vi "XYZ-2.vi"() -> ()   [LabVIEW 2010]
uses:
  <vilib>/Utility/error.llb/DialogType.ctl
  <vilib>/DAQmx/write.llb/DAQmx Write (Analog DBL 1Chan 1Samp).vi
  <vilib>/DAQmx/create/channels.llb/DAQmx Create Channel (AO-Voltage-Basic).vi
  <vilib>/daqmx/miscellaneous.llb/DAQmx Fill In Error Info.vi
  Instance           2 20Saved   XYZ 3.6.2.01 .vi
  Instance           5 20Saved   XYZ 3.6.2.01 .vi
  Instance           7 20Saved   XYZ 3.6.2.01 .vi
  Instance           8 20Saved   XYZ 3.6.2.01 .vi
  <vilib>/Utility/file.llb/Write To Spreadsheet File (DBL).vi
  Instance          10 20Saved   XYZ 3.6.2.01 .vi
  Instance          14 20Saved   XYZ 3.6.2.01 .vi
  Instance          11 20Saved   XYZ 3.6.2.01 .vi
  <vilib>/measure/NI_MABase.lvlib
panel:
  in  "save":bool
  out "pos Z":dbl=100.0
  in  "Return Z":bool
  out "Pos Z inv":dbl
  in  "Go to Z":dbl
  in  "R Z":bool
  out "?":bool
  in  "# steps z":dbl
  in  "Amp inv Z":dbl=2.0
  out "Pos Y inv":dbl
  out "Pos z":dbl=1.0
  in  "Max Z":dbl=1.0
  in  "Ampl Z":dbl=2.0
  in  "R Y":bool
  out "?":bool
  in  "Ampl Y Inv":dbl=2.5
  in  "# steps Y":dbl
  out "Pos Y inv":dbl
  out "Pos Y":dbl=1.0
  in  "Max Y":dbl=1.0
  in  "Ampl Y":dbl=2.5
  in  "R X":bool
  out "?":bool
  in  "Ampl X Inv":dbl=2.5
  in  "# steps x":dbl
  out "Pos X inv":dbl
  out "Pos X":dbl=1.0
  in  "Max X":dbl=1.0
  in  "Ampl X":dbl=2.5
  out "?":bool=TRUE
  out "?":bool=TRUE
  in  "Forward":bool=TRUE
  in  "Return Y":bool
  out "pos Y INV":dbl
  in  "Go to Y":dbl
  out "pos Y":dbl=100.0
  in  "Return X":bool
  out "pos X":dbl=100.0
  out "Pos X INV":dbl=543.0
  in  "Go to X":dbl
  in  "MAIN":path=path "C:/Users/John Markert/Desktop/main data.lvm"
  in  "?":bool
  out "Data":dbl[][](array[numeric])=[[0.0, 0.0, 0.0, 4.53e-05, 0.0]]
  out "Matrix 5 x":dbl=1.0
  # "[X,R]"
  # "[Y,0]"
  # "Y"
  # "Z"
  # "X"
  # "Max _ # of groupings\nof # of steps pulses each"
  # "Backwards"
  # "Lock-in ON"
  # "DC Volt ON"
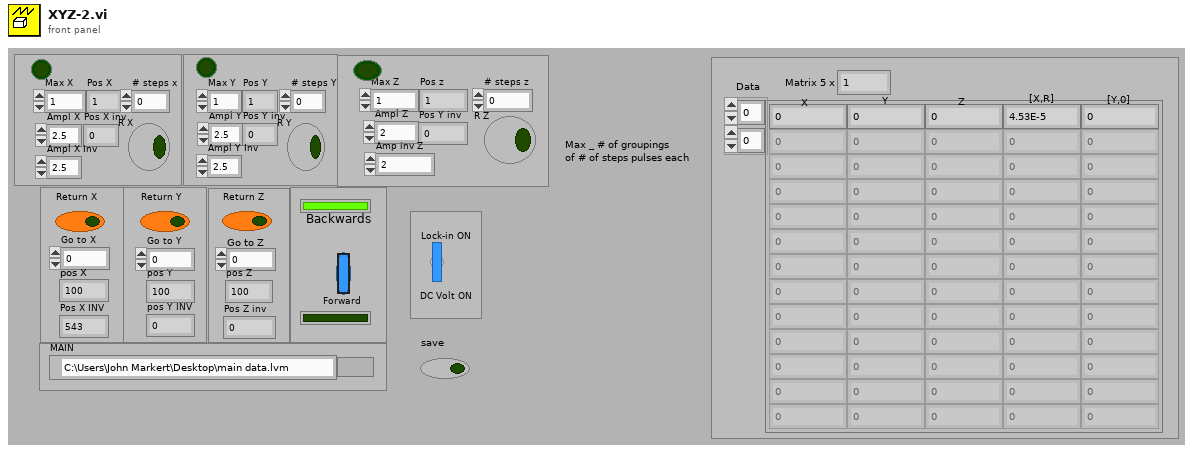
[diagram p1: front panel]
types:
  T1 = typedef "DialogType.ctl" = u16
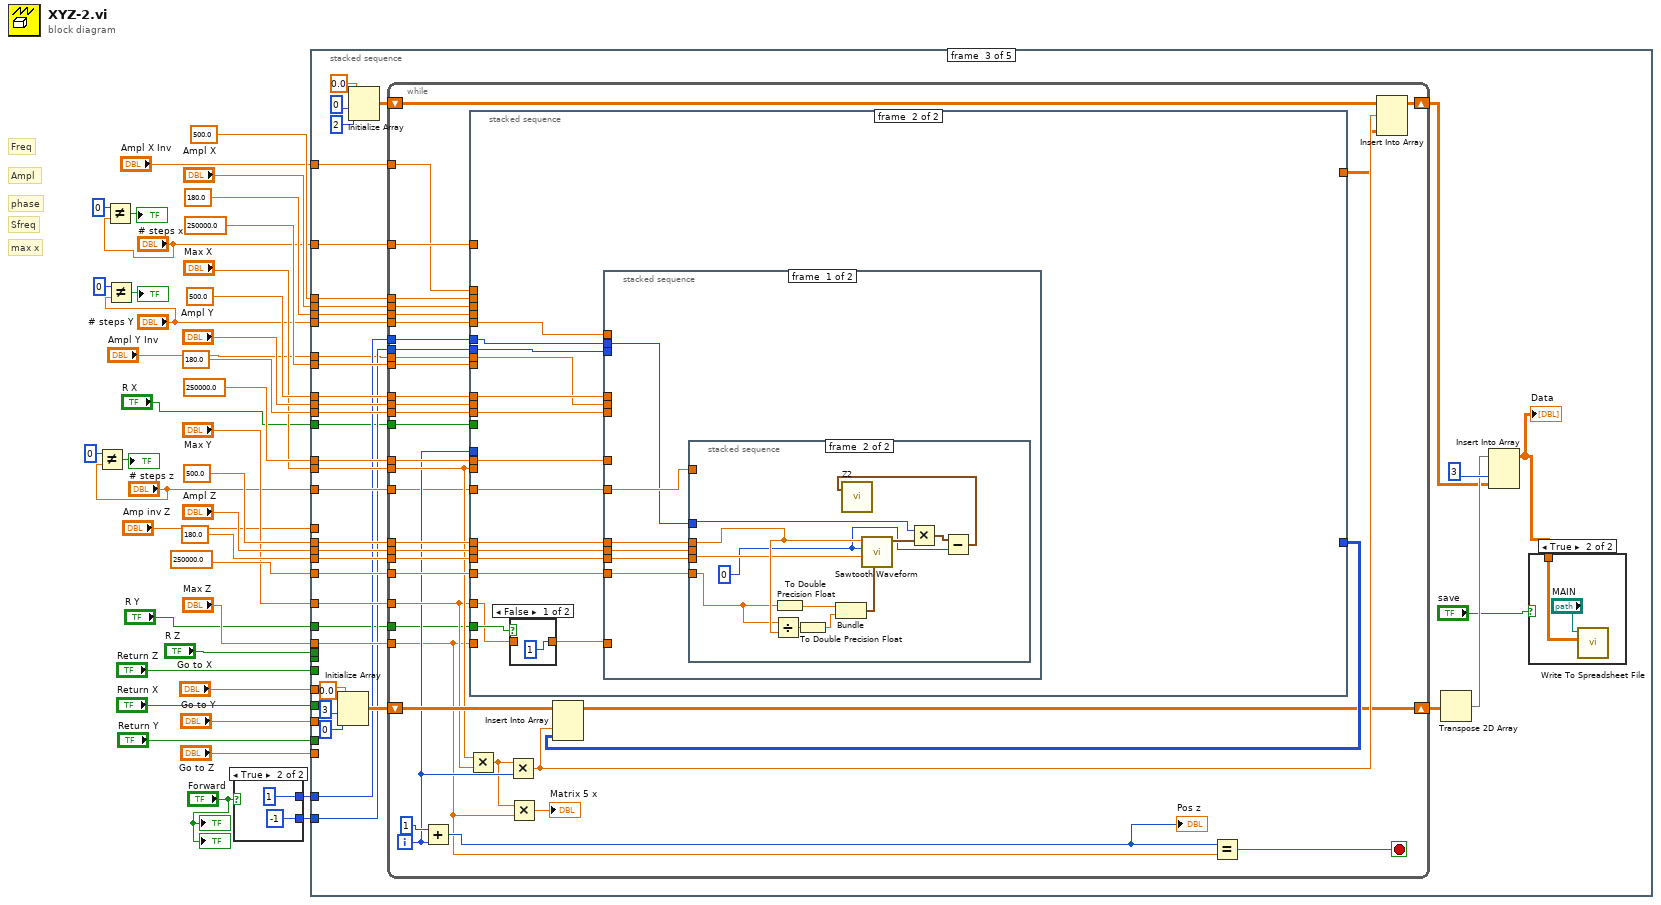
[diagram p0: block diagram]
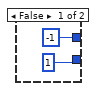
[diagram p2: hidden frame]
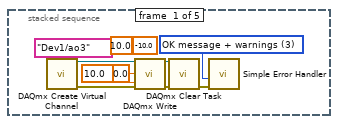
[diagram p3: hidden frame]
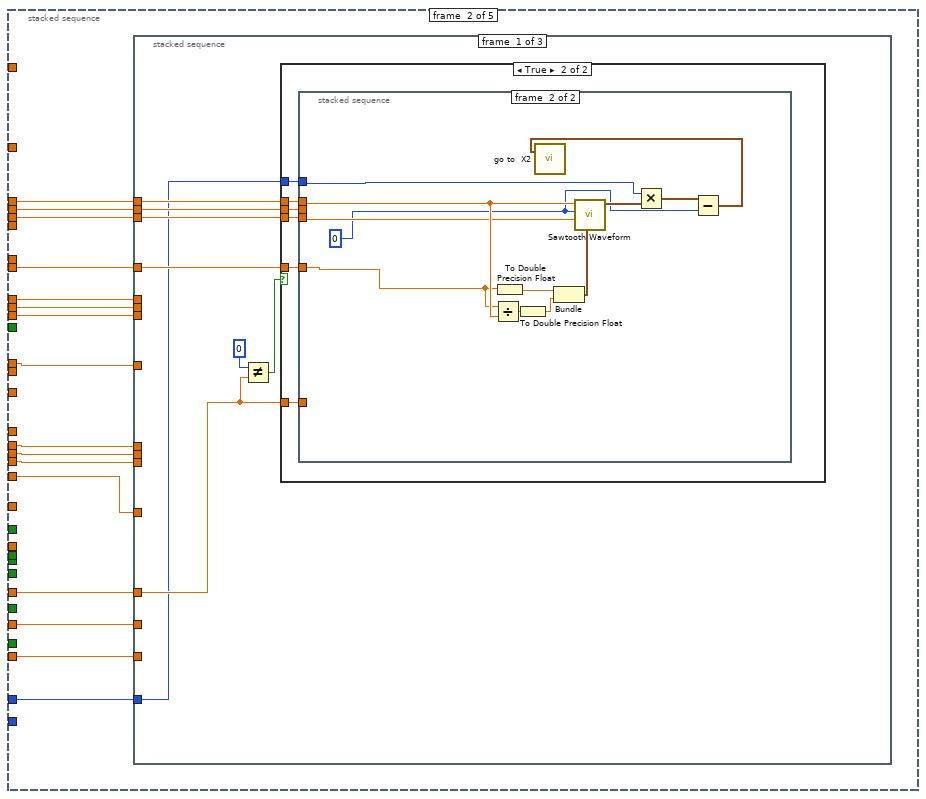
[diagram p4: hidden frame]
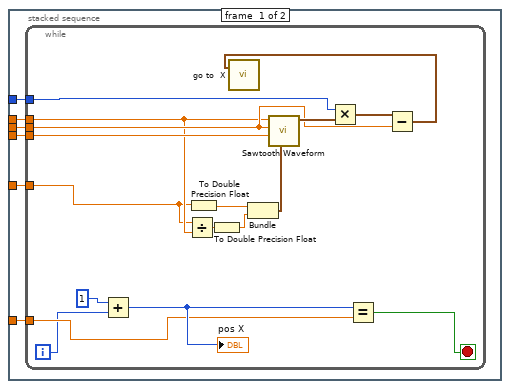
[diagram p6: hidden frame]
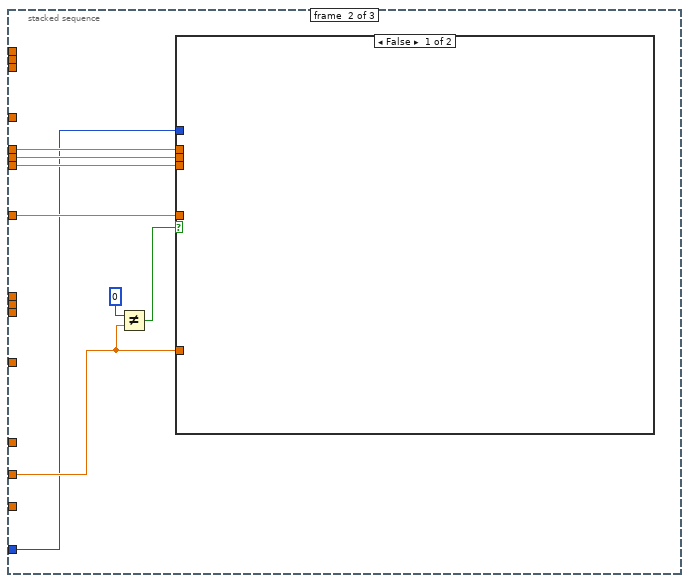
[diagram p7: hidden frame]
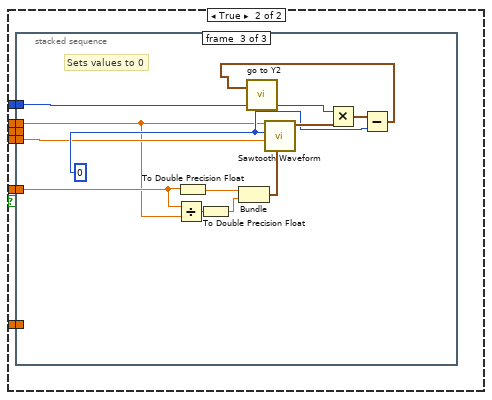
[diagram p8: hidden frame]
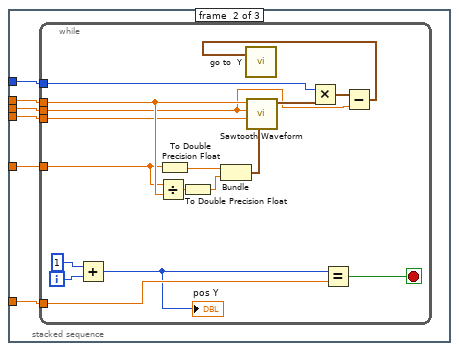
[diagram p10: hidden frame]
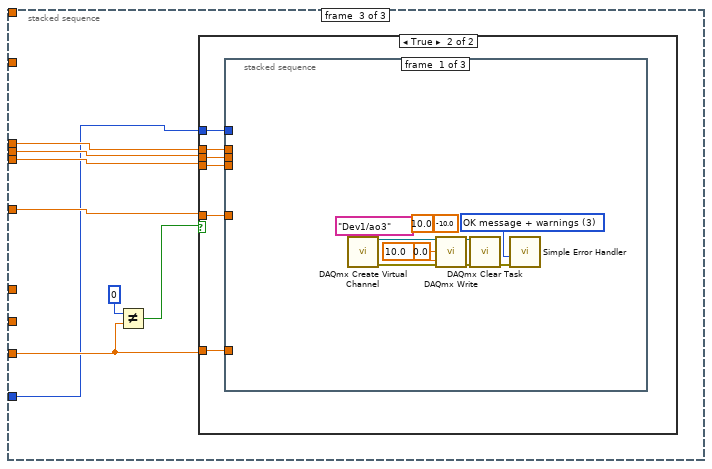
[diagram p11: hidden frame]
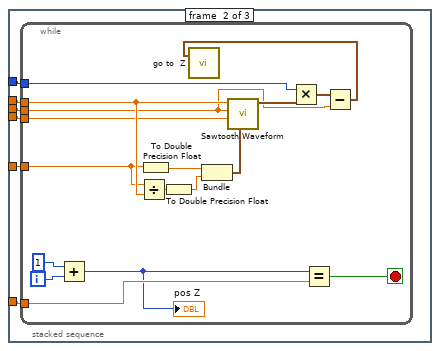
[diagram p13: hidden frame]
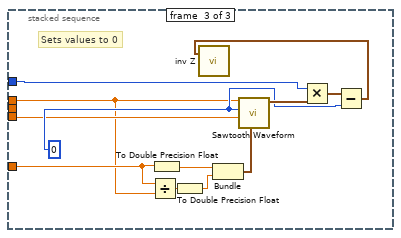
[diagram p14: hidden frame]
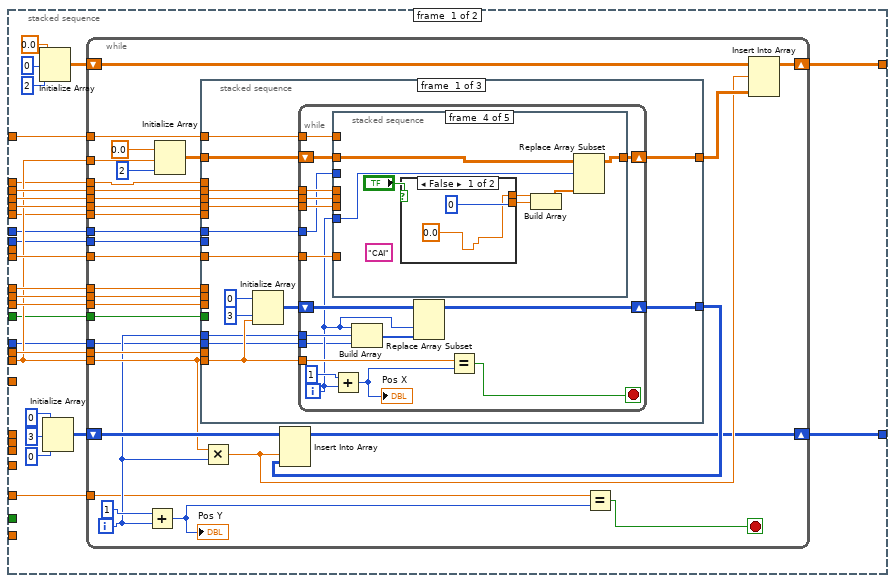
[diagram p16: hidden frame]
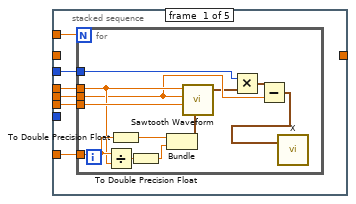
[diagram p17: hidden frame]
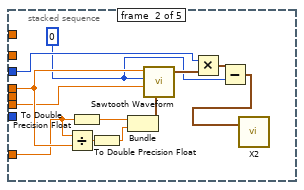
[diagram p18: hidden frame]
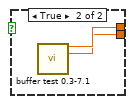
[diagram p20: hidden frame]
diagram:
  # "max x"
  # "Sfreq"
  # "phase"
  # "Ampl"
  # "Freq"
  n1 = Not Equal?(x=0, y="# steps z") -> (x != y?=→"?":bool)
  n2 = Not Equal?(x=0, y="# steps x") -> (x != y?=→"?":bool)
  n3 = Not Equal?(x=0, y="# steps Y") -> (x != y?=→"?":bool)
  n4 = case shown="True" "Forward" {
    tunnel: [-1 1] -> w21
    tunnel: [1 -1] -> w20
    frame False {
    }
    frame True {
    }
  }
  n5 = stacked-sequence {
    tunnel: 500.0 ("Freq X") -> [_ w70 w266 _ w706]
    tunnel: "Ampl X" -> [_ w69 w265 _ w705]
    tunnel: 180.0 ("Phase X") -> [_ w68 w264 _ w704]
    tunnel: 250000.0 ("S. Freq X") -> [_ w67 w263 _ w703]
    tunnel: 500.0 ("Freq Y") -> [_ w66 w262 _ w701]
    tunnel: "Ampl Y" -> [_ w65 w261 _ w700]
    tunnel: 180.0 ("Phase Y") -> [_ w64 w260 _ w699]
    tunnel: 250000.0 ("S. Freq Y") -> [_ w63 w259 w639 w698]
    tunnel: "Max X" -> [_ _ w258 _ _]
    tunnel: "Max Y" -> [_ _ w257 _ w693]
    tunnel: 500.0 ("Freq Z") -> [_ w62 w256 w633 w696]
    tunnel: "Ampl Z" -> [_ w61 w255 _ w695]
    tunnel: 180.0 ("Phase Z") -> [_ w60 w254 w640 w694]
    tunnel: 250000.0 ("S. Freq Z") -> [_ w59 w253 _ w691]
    tunnel: "Max Z" -> [_ _ w252 w635 _]
    tunnel: "Go to X" -> [_ w58 _ _ w702]
    tunnel: "Go to Y" -> [_ w57 _ _ w697]
    tunnel: "Go to Z" -> [_ w56 _ _ w692]
    tunnel: "# steps x" -> [_ _ w239 _ _]
    tunnel: "# steps Y" -> [_ _ w238 _ _]
    tunnel: "# steps z" -> [_ _ w237 w638 _]
    tunnel: w21 -> [_ w55 w236 _ w690]
    tunnel: w20 -> [_ _ w235 w637 w689]
    tunnel: "Return Z" -> [_ _ _ _ w688]
    tunnel: "Return X" -> [_ _ _ _ w687]
    tunnel: "Return Y" -> [_ _ _ _ w686]
    tunnel: "Ampl X Inv" -> [_ _ w234 _ _]
    tunnel: "Ampl Y Inv" -> [_ _ w233 _ _]
    tunnel: "Amp inv Z" -> [_ _ _ w634 _]
    tunnel: "R X" -> [_ _ w232 _ _]
    tunnel: "R Y" -> [_ _ w231 _ _]
    tunnel: [_ _ _ w632 _] -> _
    tunnel: "R Z" -> [_ _ _ w632 _]
    frame #0 {
      w47 = T1 3 items=["no dialog", "OK message", "continue or stop message", "OK message + warnings", "continue/stop + warnings"] ("type of dialog (OK msg:1)")
      n6 = call-poly <vilib>:"DAQmx Create Virtual Channel.vi"("maximum value"=10.0 ("Maximum Value"), "minimum value"=-10.0 ("Minimum Value"), "physical channels"=tag "Dev1/ao3" ("Physical Channel")) -> ("task out"=w50:refnum<k21>, "error out"=w51:errorcluster)  [unwired: 6 in, 5 out]
      n7 = call-poly <vilib>:"DAQmx Write.vi"("task/channels in"=w50, "data"=0.0 ("Voltage Output"), "timeout"=10.0, "error in"=w51) -> ("task out"=w45:refnum<k21>, "error out"=w46:errorcluster)  [unwired: 1 in, 9 out]
      n8 = call <vilib>:"DAQmx Clear Task.vi"("task in"=w45, "error in"=w46) -> ("error out"=w44:errorcluster)  [unwired: 13 out]
      n9 = call <vilib>:"Simple Error Handler.vi"("type of dialog (OK msg:1)"=w47, "error in (no error)"=w44) -> ()  [unwired: 8 out]
    }
    frame #1 {
      n10 = stacked-sequence {
        tunnel: w70 -> [w78 _ _]
        tunnel: w69 -> [w77 _ _]
        tunnel: w68 -> [w76 _ _]
        tunnel: w67 -> [w75 _ _]
        tunnel: w66 -> [_ w125 _]
        tunnel: w65 -> [_ w124 _]
        tunnel: w64 -> [_ w123 _]
        tunnel: w63 -> [_ w122 _]
        tunnel: w62 -> [_ _ w170]
        tunnel: w61 -> [_ _ w171]
        tunnel: w60 -> [_ _ w172]
        tunnel: w59 -> [_ _ w173]
        tunnel: w58 -> [w72 _ _]
        tunnel: w57 -> [_ w121 _]
        tunnel: w56 -> [_ _ w175]
        tunnel: w55 -> [w71 w120 w169]
        frame #0 {
          n11 = Not Equal?(x=0, y=w72) -> (x != y?=w74:bool)
          n12 = case shown="True" w74 {
            tunnel: w78 -> [_ w81]
            tunnel: w77 -> [_ w82]
            tunnel: w76 -> [_ w84]
            tunnel: w75 -> [_ w80]
            tunnel: w72 -> [_ w79]
            tunnel: w71 -> [_ w83]
            frame False {
            }
            frame True {
              n13 = stacked-sequence {
                tunnel: w84 -> [w90 w110]
                tunnel: w83 -> [w89 w112]
                tunnel: w82 -> [w88 _]
                tunnel: w81 -> [w87 w111]
                tunnel: w80 -> [w86 w109]
                tunnel: w79 -> [w85 _]
                frame #0 {
                  n14 = while {
                    tunnel: w90 -> [w107]
                    tunnel: w89 -> [w106]
                    tunnel: w88 -> [w102]
                    tunnel: w87 -> [w98]
                    tunnel: w86 -> [w97]
                    tunnel: w85 -> [w92]
                    i -> [w91]
                    stop <- w93 stop-if-true
                    n15 = Add(x=1, y=w91) -> (x+y=w94:i32)
                    "pos X" <- w94
                    n16 = Divide(x=w97, y=w98) -> (x/y=w101:dbl)
                    n17 = To Double Precision Float(number=w97) -> (double precision float=w100:dbl)
                    n18 = To Double Precision Float(number=w101) -> (double precision float=w99:dbl)
                    n19 = Bundle(w100, w99) -> (w96:cluster{dbl, dbl})  [unwired: 1 out]
                    n20 = call <vilib>:"Sawtooth Waveform.vi"("sampling info"=w96, "phase"=w107, "amplitude"=w102, "frequency"=w98) -> ("signal out"=w105:waveform(dbl))  [unwired: 3 in, 4 out]
                    n21 = Multiply(x=w106, y=w105) -> (x*y=w104:waveform(dbl))
                    n22 = Equal?(x=w94, y=w92) -> (x = y?=w93:bool)
                    n23 = Subtract(x=w104, y=w102) -> (x-y=w103:waveform(dbl))
                    n24 = call "go to  X"("data"=w103) -> ()  [unwired: 5 in, 14 out]
                  }
                }
                frame #1 {
                  w108 = 0
                  n25 = Divide(x=w109, y=w111) -> (x/y=w116:dbl)
                  n26 = To Double Precision Float(number=w109) -> (double precision float=w115:dbl)
                  n27 = To Double Precision Float(number=w116) -> (double precision float=w114:dbl)
                  n28 = Bundle(w115, w114) -> (w113:cluster{dbl, dbl})  [unwired: 1 out]
                  n29 = call <vilib>:"Sawtooth Waveform.vi"("sampling info"=w113, "phase"=w110, "amplitude"=w108, "frequency"=w111) -> ("signal out"=w119:waveform(dbl))  [unwired: 3 in, 4 out]
                  n30 = Multiply(x=w112, y=w119) -> (x*y=w118:waveform(dbl))
                  n31 = Subtract(x=w118, y=w108) -> (x-y=w117:waveform(dbl))
                  n32 = call "go to  X2"("data"=w117) -> ()  [unwired: 5 in, 14 out]
                }
              }
            }
          }
        }
        frame #1 {
          n33 = Not Equal?(x=0, y=w121) -> (x != y?=w127:bool)
          n34 = case shown="False" w127 {
            tunnel: w125 -> [_ w133]
            tunnel: w124 -> [_ w132]
            tunnel: w123 -> [_ w131]
            tunnel: w122 -> [_ w130]
            tunnel: w121 -> [_ w129]
            tunnel: w120 -> [_ w128]
            frame False {
            }
            frame True {
              n35 = stacked-sequence {
                tunnel: w133 -> [_ w139 w158]
                tunnel: w132 -> [_ w138 _]
                tunnel: w131 -> [_ w137 w160]
                tunnel: w130 -> [_ w136 w159]
                tunnel: w129 -> [_ w135 _]
                tunnel: w128 -> [_ w134 w162]
                frame #0 {
                }
                frame #1 {
                  n36 = while {
                    tunnel: w139 -> [w150]
                    tunnel: w138 -> [w142]
                    tunnel: w137 -> [w149]
                    tunnel: w136 -> [w148]
                    tunnel: w135 -> [w146]
                    tunnel: w134 -> [w143]
                    i -> [w151]
                    stop <- w147 stop-if-true
                    n37 = Add(x=1, y=w151) -> (x+y=w145:i32)
                    "pos Y" <- w145
                    n38 = Divide(x=w148, y=w150) -> (x/y=w156:dbl)
                    n39 = To Double Precision Float(number=w148) -> (double precision float=w154:dbl)
                    n40 = To Double Precision Float(number=w156) -> (double precision float=w153:dbl)
                    n41 = Bundle(w154, w153) -> (w155:cluster{dbl, dbl})  [unwired: 1 out]
                    n42 = call <vilib>:"Sawtooth Waveform.vi"("sampling info"=w155, "phase"=w149, "amplitude"=w142, "frequency"=w150) -> ("signal out"=w144:waveform(dbl))  [unwired: 3 in, 4 out]
                    n43 = Multiply(x=w143, y=w144) -> (x*y=w141:waveform(dbl))
                    n44 = Equal?(x=w145, y=w146) -> (x = y?=w147:bool)
                    n45 = Subtract(x=w141, y=w142) -> (x-y=w140:waveform(dbl))
                    n46 = call "go to  Y"("data"=w140) -> ()  [unwired: 5 in, 14 out]
                  }
                }
                frame #2 {
                  w161 = 0
                  # "Sets values to 0"
                  n47 = Divide(x=w159, y=w158) -> (x/y=w168:dbl)
                  n48 = To Double Precision Float(number=w159) -> (double precision float=w166:dbl)
                  n49 = To Double Precision Float(number=w168) -> (double precision float=w165:dbl)
                  n50 = Bundle(w166, w165) -> (w167:cluster{dbl, dbl})  [unwired: 1 out]
                  n51 = call <vilib>:"Sawtooth Waveform.vi"("sampling info"=w167, "phase"=w160, "amplitude"=w161, "frequency"=w158) -> ("signal out"=w164:waveform(dbl))  [unwired: 3 in, 4 out]
                  n52 = Multiply(x=w162, y=w164) -> (x*y=w163:waveform(dbl))
                  n53 = Subtract(x=w163, y=w161) -> (x-y=w157:waveform(dbl))
                  n54 = call "go to Y2"("data"=w157) -> ()  [unwired: 5 in, 14 out]
                }
              }
            }
          }
        }
        frame #2 {
          n55 = Not Equal?(x=0, y=w175) -> (x != y?=w174:bool)
          n56 = case shown="True" w174 {
            tunnel: w170 -> [_ w182]
            tunnel: w171 -> [_ w181]
            tunnel: w172 -> [_ w180]
            tunnel: w173 -> [_ w179]
            tunnel: w175 -> [_ w178]
            tunnel: w169 -> [_ w177]
            frame False {
            }
            frame True {
              n57 = stacked-sequence {
                tunnel: w182 -> [_ w199 w217]
                tunnel: w181 -> [_ w198 _]
                tunnel: w180 -> [_ w197 w219]
                tunnel: w179 -> [_ w196 w218]
                tunnel: w178 -> [_ w195 _]
                tunnel: w177 -> [_ w194 w221]
                frame #0 {
                  w186 = T1 3 items=["no dialog", "OK message", "continue or stop message", "OK message + warnings", "continue/stop + warnings"] ("type of dialog (OK msg:1)")
                  n58 = call-poly <vilib>:"DAQmx Create Virtual Channel.vi"("maximum value"=10.0 ("Maximum Value"), "minimum value"=-10.0 ("Minimum Value"), "physical channels"=tag "Dev1/ao3" ("Physical Channel")) -> ("task out"=w189:refnum<k21>, "error out"=w190:errorcluster)  [unwired: 6 in, 5 out]
                  n59 = call-poly <vilib>:"DAQmx Write.vi"("task/channels in"=w189, "data"=0.0 ("Voltage Output"), "timeout"=10.0, "error in"=w190) -> ("task out"=w184:refnum<k21>, "error out"=w185:errorcluster)  [unwired: 1 in, 9 out]
                  n60 = call <vilib>:"DAQmx Clear Task.vi"("task in"=w184, "error in"=w185) -> ("error out"=w183:errorcluster)  [unwired: 13 out]
                  n61 = call <vilib>:"Simple Error Handler.vi"("type of dialog (OK msg:1)"=w186, "error in (no error)"=w183) -> ()  [unwired: 8 out]
                }
                frame #1 {
                  n62 = while {
                    tunnel: w199 -> [w210]
                    tunnel: w198 -> [w201]
                    tunnel: w197 -> [w209]
                    tunnel: w196 -> [w208]
                    tunnel: w195 -> [w206]
                    tunnel: w194 -> [w203]
                    i -> [w211]
                    stop <- w207 stop-if-true
                    n63 = Add(x=1, y=w211) -> (x+y=w205:i32)
                    "pos Z" <- w205
                    n64 = Divide(x=w208, y=w210) -> (x/y=w216:dbl)
                    n65 = To Double Precision Float(number=w208) -> (double precision float=w214:dbl)
                    n66 = To Double Precision Float(number=w216) -> (double precision float=w213:dbl)
                    n67 = Bundle(w214, w213) -> (w215:cluster{dbl, dbl})  [unwired: 1 out]
                    n68 = call <vilib>:"Sawtooth Waveform.vi"("sampling info"=w215, "phase"=w209, "amplitude"=w201, "frequency"=w210) -> ("signal out"=w204:waveform(dbl))  [unwired: 3 in, 4 out]
                    n69 = Multiply(x=w203, y=w204) -> (x*y=w200:waveform(dbl))
                    n70 = Equal?(x=w205, y=w206) -> (x = y?=w207:bool)
                    n71 = Subtract(x=w200, y=w201) -> (x-y=w202:waveform(dbl))
                    n72 = call "go to  Z"("data"=w202) -> ()  [unwired: 5 in, 14 out]
                  }
                }
                frame #2 {
                  w220 = 0
                  # "Sets values to 0"
                  n73 = Divide(x=w218, y=w217) -> (x/y=w228:dbl)
                  n74 = To Double Precision Float(number=w218) -> (double precision float=w226:dbl)
                  n75 = To Double Precision Float(number=w228) -> (double precision float=w225:dbl)
                  n76 = Bundle(w226, w225) -> (w227:cluster{dbl, dbl})  [unwired: 1 out]
                  n77 = call <vilib>:"Sawtooth Waveform.vi"("sampling info"=w227, "phase"=w219, "amplitude"=w220, "frequency"=w217) -> ("signal out"=w224:waveform(dbl))  [unwired: 3 in, 4 out]
                  n78 = Multiply(x=w221, y=w224) -> (x*y=w222:waveform(dbl))
                  n79 = Subtract(x=w222, y=w220) -> (x-y=w223:waveform(dbl))
                  n80 = call "inv Z"("data"=w223) -> ()  [unwired: 5 in, 14 out]
                }
              }
            }
          }
        }
      }
    }
    frame #2 {
      n81 = Initialize Array(0.0, 3, 0) -> (w247:dbl[][])
      n82 = Initialize Array(0.0, 0, 2) -> (w246:dbl[][])
      n83 = while {
        tunnel: w266 -> [w305]
        tunnel: w265 -> [w304]
        tunnel: w264 -> [w303]
        tunnel: w263 -> [w302]
        tunnel: w262 -> [w301]
        tunnel: w261 -> [w300]
        tunnel: w260 -> [w299]
        tunnel: w259 -> [w298]
        tunnel: w258 -> [w288]
        tunnel: w257 -> [w286]
        tunnel: w256 -> [w297]
        tunnel: w255 -> [w296]
        tunnel: w254 -> [w295]
        tunnel: w253 -> [w294]
        tunnel: w252 -> [w283]
        shift-right: [w275] -> w244
        shift-left: w247 -> [w293]
        shift-right: [w274] -> w240
        shift-left: w246 -> [w290]
        tunnel: w239 -> [w280]
        tunnel: w238 -> [w279]
        tunnel: w237 -> [w278]
        tunnel: w236 -> [w277]
        tunnel: w235 -> [w276]
        tunnel: w234 -> [w272]
        tunnel: w233 -> [w271]
        tunnel: w232 -> [w270]
        tunnel: w231 -> [w269]
        i -> [w285]
        stop <- w291 stop-if-true
        n84 = Add(x=1, y=w285) -> (x+y=w287:i32)
        "Pos z" <- w287
        n85 = Multiply(x=w288, y=w286) -> (x*y=w282:dbl)
        n86 = stacked-sequence {
          tunnel: w305 -> [w332 _]
          tunnel: w304 -> [w331 _]
          tunnel: w303 -> [w330 _]
          tunnel: w302 -> [w329 _]
          tunnel: w301 -> [w328 w539]
          tunnel: w300 -> [w327 _]
          tunnel: w299 -> [w326 w538]
          tunnel: w298 -> [w325 w537]
          tunnel: w288 -> [w324 _]
          tunnel: w286 -> [w319 w530]
          tunnel: w297 -> [_ w543]
          tunnel: w296 -> [_ w542]
          tunnel: w295 -> [_ w541]
          tunnel: w294 -> [_ w540]
          tunnel: w283 -> [_ _]
          tunnel: [w308 _] -> w292
          tunnel: w285 -> [w314 _]
          tunnel: [w309 _] -> w273
          tunnel: w280 -> [w313 _]
          tunnel: w279 -> [w312 w536]
          tunnel: w278 -> [_ w535]
          tunnel: w277 -> [w311 w534]
          tunnel: w276 -> [w310 w533]
          tunnel: w272 -> [w307 _]
          tunnel: w271 -> [_ w532]
          tunnel: w270 -> [w306 _]
          tunnel: w269 -> [_ w531]
          frame #0 {
            n87 = Initialize Array(0.0, 0, 2) -> (w315:dbl[][])
            n88 = Initialize Array(0, 3, 0) -> (w320:i32[][])
            n89 = while {
              tunnel: w332 -> [w364]
              tunnel: w331 -> [w363]
              tunnel: w330 -> [w362]
              tunnel: w329 -> [w361]
              tunnel: w324 -> [w350]
              tunnel: w328 -> [w358]
              tunnel: w327 -> [w357]
              tunnel: w326 -> [w356]
              tunnel: w325 -> [w355]
              tunnel: w324 -> [w354]
              shift-right: [w335] -> w308
              shift-left: w320 -> [w352]
              tunnel: w319 -> [w346]
              shift-right: [w336] -> w309
              shift-left: w315 -> [w344]
              tunnel: w314 -> [w342]
              tunnel: w313 -> [w340]
              tunnel: w312 -> [w339]
              tunnel: w311 -> [w338]
              tunnel: w310 -> [w337]
              tunnel: w307 -> [w334]
              tunnel: w306 -> [w333]
              i -> [w348]
              stop <- w347 stop-if-true
              n90 = Add(x=1, y=w348) -> (x+y=w345:i32)
              "Pos Y" <- w345
              n91 = Initialize Array(0.0, w354, 2) -> (w359:dbl[][])
              n92 = stacked-sequence {
                tunnel: w364 -> [w379 _ w480]
                tunnel: w363 -> [w378 _ _]
                tunnel: w362 -> [w377 _ w483]
                tunnel: w361 -> [w376 _ w482]
                tunnel: w350 -> [w372 _ w478]
                tunnel: w359 -> [w375 _ _]
                tunnel: [w365 _ _] -> w343
                tunnel: w358 -> [_ w444 _]
                tunnel: w357 -> [_ w443 _]
                tunnel: w356 -> [_ w442 _]
                tunnel: w355 -> [_ w441 _]
                tunnel: [w366 _ _] -> w349
                tunnel: w348 -> [w370 _ _]
                tunnel: w342 -> [w369 _ _]
                tunnel: w340 -> [w368 _ w475]
                tunnel: w339 -> [_ w440 _]
                tunnel: w338 -> [w367 w439 _]
                tunnel: w337 -> [_ _ w481]
                tunnel: w334 -> [_ _ w479]
                tunnel: w333 -> [_ _ w476]
                frame #0 {
                  n93 = Initialize Array(0, 3, w372) -> (w371:i32[][])
                  n94 = while {
                    tunnel: w379 -> [w397]
                    tunnel: w378 -> [w396]
                    tunnel: w377 -> [w395]
                    tunnel: w376 -> [w394]
                    tunnel: w372 -> [w392]
                    shift-right: [w389] -> w365
                    shift-left: w375 -> [w390]
                    shift-right: [w387] -> w366
                    shift-left: w371 -> [w388]
                    tunnel: w370 -> [w384]
                    tunnel: w369 -> [w380]
                    tunnel: w368 -> [w382]
                    tunnel: w367 -> [w381]
                    i -> [w383]
                    stop <- w391 stop-if-true
                    n95 = stacked-sequence {
                      tunnel: w397 -> [w401 w419 _ _ _]
                      tunnel: w396 -> [w400 _ _ _ _]
                      tunnel: w395 -> [w403 w418 _ _ _]
                      tunnel: w394 -> [w402 w417 _ _ _]
                      tunnel: w383 -> [_ _ _ w431 _]
                      tunnel: w390 -> [_ _ _ w434 _]
                      tunnel: [_ _ _ w433 _] -> w389
                      tunnel: w382 -> [w398 _ _ _ _]
                      tunnel: w381 -> [w399 w420 _ _ _]
                      frame #0 {
                        n96 = for {
                          N: w398 -> [_]
                          tunnel: w403 -> [w415]
                          tunnel: w402 -> [w414]
                          tunnel: w401 -> [w413]
                          tunnel: w400 -> [w412]
                          tunnel: w399 -> [w411]
                          n97 = Divide(x=w414, y=w413) -> (x/y=w410:dbl)
                          n98 = To Double Precision Float(number=w414) -> (double precision float=w408:dbl)
                          n99 = To Double Precision Float(number=w410) -> (double precision float=w407:dbl)
                          n100 = Bundle(w408, w407) -> (w409:cluster{dbl, dbl})  [unwired: 1 out]
                          n101 = call <vilib>:"Sawtooth Waveform.vi"("sampling info"=w409, "phase"=w415, "amplitude"=w412, "frequency"=w413) -> ("signal out"=w405:waveform(dbl))  [unwired: 3 in, 4 out]
                          n102 = Multiply(x=w411, y=w405) -> (x*y=w406:waveform(dbl))
                          n103 = Subtract(x=w406, y=w412) -> (x-y=w404:waveform(dbl))
                          n104 = call "X"("data"=w404) -> ()  [unwired: 5 in, 14 out]
                        }
                      }
                      frame #1 {
                        w416 = 0
                        n105 = Divide(x=w417, y=w419) -> (x/y=w427:dbl)
                        n106 = To Double Precision Float(number=w417) -> (double precision float=w425:dbl)
                        n107 = To Double Precision Float(number=w427) -> (double precision float=w424:dbl)
                        n108 = Bundle(w425, w424) -> (w426:cluster{dbl, dbl})  [unwired: 1 out]
                        n109 = call <vilib>:"Sawtooth Waveform.vi"("sampling info"=w426, "phase"=w418, "amplitude"=w416, "frequency"=w419) -> ("signal out"=w422:waveform(dbl))  [unwired: 3 in, 4 out]
                        n110 = Multiply(x=w420, y=w422) -> (x*y=w423:waveform(dbl))
                        n111 = Subtract(x=w423, y=w416) -> (x-y=w421:waveform(dbl))
                        n112 = call "X2"("data"=w421) -> ()  [unwired: 5 in, 14 out]
                      }
                      frame #2 {
                      }
                      frame #3 {
                        (unwired) "CAI"
                        n113 = case shown="False" "?" {
                          tunnel: [0.0 w438] -> w430
                          tunnel: [0 w437] -> w429
                          frame False {
                          }
                          frame True {
                            n114 = call "buffer test 0.3-7.1.vi"() -> ("[X,R]"=w438:dbl, "[Y,0]"=w437:dbl)  [unwired: 14 out]
                          }
                        }
                        n115 = Build Array(w430, w429) -> (w428:dbl[])
                        n116 = Replace Array Subset(array=w434, new element=w428, index (row)=w431) -> (w433:dbl[][])  [unwired: 1 in]
                      }
                      frame #4 {
                      }
                    }
                    n117 = Add(x=1, y=w383) -> (x+y=w385:i32)
                    "Pos X" <- w385
                    n118 = Build Array(w383, w384, w380) -> (w386:i32[])
                    n119 = Replace Array Subset(array=w388, new element=w386, index (col)=w383) -> (w387:i32[][])  [unwired: 1 in]
                    n120 = Equal?(x=w392, y=w385) -> (x = y?=w391:bool)
                  }
                }
                frame #1 {
                  n121 = stacked-sequence {
                    tunnel: w444 -> [w450 w467]
                    tunnel: w443 -> [w449 _]
                    tunnel: w442 -> [w448 w466]
                    tunnel: w441 -> [w447 w465]
                    tunnel: w440 -> [w445 _]
                    tunnel: w439 -> [w446 w468]
                    frame #0 {
                      n122 = for {
                        N: w445 -> [_]
                        tunnel: w450 -> [w462]
                        tunnel: w449 -> [w461]
                        tunnel: w448 -> [w460]
                        tunnel: w447 -> [w459]
                        tunnel: w446 -> [w458]
                        n123 = Divide(x=w459, y=w462) -> (x/y=w457:dbl)
                        n124 = To Double Precision Float(number=w459) -> (double precision float=w455:dbl)
                        n125 = To Double Precision Float(number=w457) -> (double precision float=w454:dbl)
                        n126 = Bundle(w455, w454) -> (w456:cluster{dbl, dbl})  [unwired: 1 out]
                        n127 = call <vilib>:"Sawtooth Waveform.vi"("sampling info"=w456, "phase"=w460, "amplitude"=w461, "frequency"=w462) -> ("signal out"=w453:waveform(dbl))  [unwired: 3 in, 4 out]
                        n128 = Multiply(x=w458, y=w453) -> (x*y=w452:waveform(dbl))
                        n129 = Subtract(x=w452, y=w461) -> (x-y=w451:waveform(dbl))
                        n130 = call "Y"("data"=w451) -> ()  [unwired: 5 in, 14 out]
                      }
                    }
                    frame #1 {
                      w464 = 0
                      n131 = Divide(x=w465, y=w467) -> (x/y=w474:dbl)
                      n132 = To Double Precision Float(number=w465) -> (double precision float=w472:dbl)
                      n133 = To Double Precision Float(number=w474) -> (double precision float=w471:dbl)
                      n134 = Bundle(w472, w471) -> (w473:cluster{dbl, dbl})  [unwired: 1 out]
                      n135 = call <vilib>:"Sawtooth Waveform.vi"("sampling info"=w473, "phase"=w466, "amplitude"=w464, "frequency"=w467) -> ("signal out"=w470:waveform(dbl))  [unwired: 3 in, 4 out]
                      n136 = Multiply(x=w468, y=w470) -> (x*y=w469:waveform(dbl))
                      n137 = Subtract(x=w469, y=w464) -> (x-y=w463:waveform(dbl))
                      n138 = call "Y2"("data"=w463) -> ()  [unwired: 5 in, 14 out]
                    }
                  }
                }
                frame #2 {
                  n139 = case shown="False" w476 {
                    tunnel: [1 w528] -> w477
                    tunnel: w478 -> [_ w528]
                    frame False {
                    }
                    frame True {
                    }
                  }
                  n140 = stacked-sequence {
                    tunnel: w483 -> [w490 w517]
                    tunnel: w482 -> [w489 w516]
                    tunnel: w475 -> [w488 _]
                    tunnel: w481 -> [w487 w519]
                    tunnel: w480 -> [w486 w518]
                    tunnel: w479 -> [w485 _]
                    tunnel: w477 -> [w484 _]
                    frame #0 {
                      n141 = while {
                        tunnel: w486 -> [w500]
                        tunnel: w485 -> [w499]
                        tunnel: w490 -> [w498]
                        tunnel: w489 -> [w497]
                        tunnel: w484 -> [w493]
                        tunnel: w488 -> [w491]
                        tunnel: w487 -> [w492]
                        i -> [w501]
                        stop <- w496 stop-if-true
                        n142 = for {
                          N: w491 -> [_]
                          tunnel: w500 -> [w514]
                          tunnel: w499 -> [w513]
                          tunnel: w498 -> [w512]
                          tunnel: w497 -> [w511]
                          tunnel: w492 -> [w510]
                          n143 = Divide(x=w511, y=w514) -> (x/y=w509:dbl)
                          n144 = To Double Precision Float(number=w511) -> (double precision float=w507:dbl)
                          n145 = To Double Precision Float(number=w509) -> (double precision float=w506:dbl)
                          n146 = Bundle(w507, w506) -> (w508:cluster{dbl, dbl})  [unwired: 1 out]
                          n147 = call <vilib>:"Sawtooth Waveform.vi"("sampling info"=w508, "phase"=w512, "amplitude"=w513, "frequency"=w514) -> ("signal out"=w505:waveform(dbl))  [unwired: 3 in, 4 out]
                          n148 = Multiply(x=w510, y=w505) -> (x*y=w504:waveform(dbl))
                          n149 = Subtract(x=w504, y=w513) -> (x-y=w503:waveform(dbl))
                          n150 = call "Inv X"("data"=w503) -> ()  [unwired: 5 in, 14 out]
                        }
                        n151 = Add(x=1, y=w501) -> (x+y=w494:i32)
                        n152 = Subtract(x=w493, y=w494) -> (x-y=→"Pos X inv":dbl)
                        n153 = Equal?(x=w494, y=w493) -> (x = y?=w496:bool)
                      }
                    }
                    frame #1 {
                      w515 = 0
                      n154 = Divide(x=w516, y=w518) -> (x/y=w526:dbl)
                      n155 = To Double Precision Float(number=w516) -> (double precision float=w524:dbl)
                      n156 = To Double Precision Float(number=w526) -> (double precision float=w523:dbl)
                      n157 = Bundle(w524, w523) -> (w525:cluster{dbl, dbl})  [unwired: 1 out]
                      n158 = call <vilib>:"Sawtooth Waveform.vi"("sampling info"=w525, "phase"=w517, "amplitude"=w515, "frequency"=w518) -> ("signal out"=w522:waveform(dbl))  [unwired: 3 in, 4 out]
                      n159 = Multiply(x=w519, y=w522) -> (x*y=w521:waveform(dbl))
                      n160 = Subtract(x=w521, y=w515) -> (x-y=w520:waveform(dbl))
                      n161 = call "Inv X2"("data"=w520) -> ()  [unwired: 5 in, 14 out]
                    }
                  }
                }
              }
              n162 = Multiply(x=w350, y=w348) -> (x*y=w341:dbl)
              n163 = Insert Into Array(array=w352, index (col)=w341, new element=w349) -> (w335:i32[][])  [unwired: 1 in]
              n164 = Equal?(x=w346, y=w345) -> (x = y?=w347:bool)
              n165 = Insert Into Array(array=w344, index (row)=w341, new element=w343) -> (w336:dbl[][])  [unwired: 1 in]
            }
          }
          frame #1 {
            n166 = case shown="False" w531 {
              tunnel: [1 w545] -> w529
              tunnel: w530 -> [_ w545]
              frame False {
              }
              frame True {
              }
            }
            n167 = stacked-sequence {
              tunnel: w543 -> [w551 _]
              tunnel: w542 -> [w550 _]
              tunnel: w541 -> [w549 _]
              tunnel: w540 -> [w548 _]
              tunnel: w529 -> [_ w588]
              tunnel: w539 -> [_ w587]
              tunnel: w532 -> [_ w586]
              tunnel: w538 -> [_ w585]
              tunnel: w537 -> [_ w584]
              tunnel: w536 -> [_ w583]
              tunnel: w535 -> [w547 _]
              tunnel: w534 -> [w546 _]
              tunnel: w533 -> [_ w582]
              frame #0 {
                n168 = stacked-sequence {
                  tunnel: w551 -> [w557 w573]
                  tunnel: w550 -> [w556 _]
                  tunnel: w549 -> [w555 w572]
                  tunnel: w548 -> [w554 w571]
                  tunnel: w547 -> [w552 _]
                  tunnel: w546 -> [w553 w574]
                  frame #0 {
                    n169 = for {
                      N: w552 -> [_]
                      tunnel: w557 -> [w569]
                      tunnel: w556 -> [w568]
                      tunnel: w555 -> [w567]
                      tunnel: w554 -> [w566]
                      tunnel: w553 -> [w565]
                      n170 = Divide(x=w566, y=w569) -> (x/y=w564:dbl)
                      n171 = To Double Precision Float(number=w566) -> (double precision float=w562:dbl)
                      n172 = To Double Precision Float(number=w564) -> (double precision float=w561:dbl)
                      n173 = Bundle(w562, w561) -> (w563:cluster{dbl, dbl})  [unwired: 1 out]
                      n174 = call <vilib>:"Sawtooth Waveform.vi"("sampling info"=w563, "phase"=w567, "amplitude"=w568, "frequency"=w569) -> ("signal out"=w560:waveform(dbl))  [unwired: 3 in, 4 out]
                      n175 = Multiply(x=w565, y=w560) -> (x*y=w559:waveform(dbl))
                      n176 = Subtract(x=w559, y=w568) -> (x-y=w558:waveform(dbl))
                      n177 = call "Z"("data"=w558) -> ()  [unwired: 4 in, 15 out]
                    }
                  }
                  frame #1 {
                    w570 = 0
                    n178 = Divide(x=w571, y=w573) -> (x/y=w581:dbl)
                    n179 = To Double Precision Float(number=w571) -> (double precision float=w579:dbl)
                    n180 = To Double Precision Float(number=w581) -> (double precision float=w578:dbl)
                    n181 = Bundle(w579, w578) -> (w580:cluster{dbl, dbl})  [unwired: 1 out]
                    n182 = call <vilib>:"Sawtooth Waveform.vi"("sampling info"=w580, "phase"=w572, "amplitude"=w570, "frequency"=w573) -> ("signal out"=w577:waveform(dbl))  [unwired: 3 in, 4 out]
                    n183 = Multiply(x=w574, y=w577) -> (x*y=w576:waveform(dbl))
                    n184 = Subtract(x=w576, y=w570) -> (x-y=w575:waveform(dbl))
                    n185 = call "Z2"("data"=w575) -> ()  [unwired: 4 in, 15 out]
                  }
                }
              }
              frame #1 {
                n186 = stacked-sequence {
                  tunnel: w588 -> [w595 _]
                  tunnel: w587 -> [w594 w624]
                  tunnel: w586 -> [w593 _]
                  tunnel: w585 -> [w592 w623]
                  tunnel: w584 -> [w591 w622]
                  tunnel: w583 -> [w590 _]
                  tunnel: w582 -> [w589 w625]
                  frame #0 {
                    n187 = while {
                      tunnel: w594 -> [w605]
                      tunnel: w593 -> [w604]
                      tunnel: w592 -> [w603]
                      tunnel: w591 -> [w602]
                      tunnel: w595 -> [w598]
                      tunnel: w590 -> [w596]
                      tunnel: w589 -> [w597]
                      i -> [w606]
                      stop <- w601 stop-if-true
                      n188 = Add(x=1, y=w606) -> (x+y=w599:i32)
                      n189 = for {
                        N: w596 -> [_]
                        tunnel: w605 -> [w619]
                        tunnel: w604 -> [w618]
                        tunnel: w603 -> [w617]
                        tunnel: w602 -> [w616]
                        tunnel: w597 -> [w615]
                        n190 = Divide(x=w616, y=w619) -> (x/y=w614:dbl)
                        n191 = To Double Precision Float(number=w616) -> (double precision float=w612:dbl)
                        n192 = To Double Precision Float(number=w614) -> (double precision float=w611:dbl)
                        n193 = Bundle(w612, w611) -> (w613:cluster{dbl, dbl})  [unwired: 1 out]
                        n194 = call <vilib>:"Sawtooth Waveform.vi"("sampling info"=w613, "phase"=w617, "amplitude"=w618, "frequency"=w619) -> ("signal out"=w609:waveform(dbl))  [unwired: 3 in, 4 out]
                        n195 = Multiply(x=w615, y=w609) -> (x*y=w610:waveform(dbl))
                        n196 = Subtract(x=w610, y=w618) -> (x-y=w608:waveform(dbl))
                        n197 = call "Inv Y"("data"=w608) -> ()  [unwired: 5 in, 14 out]
                      }
                      n198 = Subtract(x=w598, y=w599) -> (x-y=→"Pos Y inv":dbl)
                      n199 = Equal?(x=w599, y=w598) -> (x = y?=w601:bool)
                    }
                  }
                  frame #1 {
                    w621 = 0
                    n200 = Divide(x=w622, y=w624) -> (x/y=w631:dbl)
                    n201 = To Double Precision Float(number=w622) -> (double precision float=w629:dbl)
                    n202 = To Double Precision Float(number=w631) -> (double precision float=w628:dbl)
                    n203 = Bundle(w629, w628) -> (w630:cluster{dbl, dbl})  [unwired: 1 out]
                    n204 = call <vilib>:"Sawtooth Waveform.vi"("sampling info"=w630, "phase"=w623, "amplitude"=w621, "frequency"=w624) -> ("signal out"=w626:waveform(dbl))  [unwired: 3 in, 4 out]
                    n205 = Multiply(x=w625, y=w626) -> (x*y=w627:waveform(dbl))
                    n206 = Subtract(x=w627, y=w621) -> (x-y=w620:waveform(dbl))
                    n207 = call "Inv 2"("data"=w620) -> ()  [unwired: 5 in, 14 out]
                  }
                }
              }
            }
          }
        }
        n208 = Multiply(x=w282, y=w285) -> (x*y=w284:dbl)
        n209 = Multiply(x=w282, y=w283) -> (x*y=→"Matrix 5 x":dbl)
        n210 = Insert Into Array(array=w293, index (col)=w284, new element=w292) -> (w275:dbl[][])  [unwired: 1 in]
        n211 = Equal?(x=w287, y=w283) -> (x = y?=w291:bool)
        n212 = Insert Into Array(array=w290, index (row)=w284, new element=w273) -> (w274:dbl[][])  [unwired: 1 in]
      }
      n213 = Transpose 2D Array(2D array=w244) -> (transposed array=w243:dbl[][])
      n214 = Insert Into Array(array=w243, index (col)=3, new element=w240) -> (w230:dbl[][])  [unwired: 1 in]
      "Data" <- w230
      n215 = case shown="True" "save" {
        tunnel: w230 -> [_ w267]
        frame False {
        }
        frame True {
          n216 = call-poly <vilib>:"Write To Spreadsheet File.vi"("2D data"=w267, "file path (dialog if empty)"="MAIN") -> ()  [unwired: 4 in, 3 out]
        }
      }
    }
    frame #3 {
      n217 = case shown="True" w632 {
        tunnel: [1 w685] -> w636
        tunnel: w635 -> [_ w685]
        frame False {
        }
        frame True {
        }
      }
      n218 = stacked-sequence {
        tunnel: w640 -> [w647 w675]
        tunnel: w639 -> [w646 w673]
        tunnel: w638 -> [w645 _]
        tunnel: w637 -> [w644 w676]
        tunnel: w636 -> [w643 _]
        tunnel: w634 -> [w642 _]
        tunnel: w633 -> [w641 w672]
        frame #0 {
          n219 = while {
            tunnel: w641 -> [w657]
            tunnel: w642 -> [w656]
            tunnel: w647 -> [w655]
            tunnel: w643 -> [w651]
            tunnel: w646 -> [w650]
            tunnel: w645 -> [w649]
            tunnel: w644 -> [w648]
            i -> [w658]
            stop <- w654 stop-if-true
            n220 = Add(x=1, y=w658) -> (x+y=w652:i32)
            n221 = for {
              N: w649 -> [_]
              tunnel: w657 -> [w667]
              tunnel: w656 -> [w666]
              tunnel: w655 -> [w665]
              tunnel: w650 -> [w662]
              tunnel: w648 -> [w661]
              n222 = Divide(x=w662, y=w667) -> (x/y=w671:dbl)
              n223 = To Double Precision Float(number=w662) -> (double precision float=w669:dbl)
              n224 = To Double Precision Float(number=w671) -> (double precision float=w668:dbl)
              n225 = Bundle(w669, w668) -> (w670:cluster{dbl, dbl})  [unwired: 1 out]
              n226 = call <vilib>:"Sawtooth Waveform.vi"("sampling info"=w670, "phase"=w665, "amplitude"=w666, "frequency"=w667) -> ("signal out"=w663:waveform(dbl))  [unwired: 3 in, 4 out]
              n227 = Multiply(x=w661, y=w663) -> (x*y=w664:waveform(dbl))
              n228 = Subtract(x=w664, y=w666) -> (x-y=w660:waveform(dbl))
              n229 = call "INV Z"("data"=w660) -> ()  [unwired: 4 in, 15 out]
            }
            n230 = Subtract(x=w651, y=w652) -> (x-y=→"Pos Y inv":dbl)
            n231 = Equal?(x=w652, y=w651) -> (x = y?=w654:bool)
          }
        }
        frame #1 {
          w674 = 0
          n232 = Divide(x=w673, y=w672) -> (x/y=w683:dbl)
          n233 = To Double Precision Float(number=w673) -> (double precision float=w681:dbl)
          n234 = To Double Precision Float(number=w683) -> (double precision float=w680:dbl)
          n235 = Bundle(w681, w680) -> (w682:cluster{dbl, dbl})  [unwired: 1 out]
          n236 = call <vilib>:"Sawtooth Waveform.vi"("sampling info"=w682, "phase"=w675, "amplitude"=w674, "frequency"=w672) -> ("signal out"=w678:waveform(dbl))  [unwired: 3 in, 4 out]
          n237 = Multiply(x=w676, y=w678) -> (x*y=w679:waveform(dbl))
          n238 = Subtract(x=w679, y=w674) -> (x-y=w677:waveform(dbl))
          n239 = call "INV Z2"("data"=w677) -> ()  [unwired: 4 in, 15 out]
        }
      }
    }
    frame #4 {
      n240 = stacked-sequence {
        tunnel: w706 -> [w715 _ _]
        tunnel: w705 -> [w714 _ _]
        tunnel: w704 -> [w713 _ _]
        tunnel: w703 -> [w712 _ _]
        tunnel: w701 -> [_ w767 _]
        tunnel: w700 -> [_ w766 _]
        tunnel: w699 -> [_ w765 _]
        tunnel: w698 -> [_ w764 _]
        tunnel: w696 -> [_ _ w802]
        tunnel: w695 -> [_ _ w801]
        tunnel: w694 -> [_ _ w800]
        tunnel: w693 -> [_ _ _]
        tunnel: w702 -> [w708 _ _]
        tunnel: w697 -> [_ w761 _]
        tunnel: w692 -> [_ _ w796]
        tunnel: w691 -> [_ _ w799]
        tunnel: w690 -> [_ _ _]
        tunnel: w689 -> [w710 w763 w798]
        tunnel: w688 -> [_ _ w795]
        tunnel: w687 -> [w709 _ _]
        tunnel: w686 -> [_ w762 _]
        frame #0 {
          n241 = case shown="True" w709 {
            tunnel: [w716 0] -> w707
            tunnel: w708 -> [w716 _]
            frame False {
            }
            frame True {
            }
          }
          n242 = Not Equal?(x=w707, y=w708) -> (x != y?=w711:bool)
          n243 = case shown="True" w711 {
            tunnel: w715 -> [_ w723]
            tunnel: w714 -> [_ w722]
            tunnel: w713 -> [_ w721]
            tunnel: w712 -> [_ w720]
            tunnel: w708 -> [_ w719]
            tunnel: w710 -> [_ w718]
            frame False {
            }
            frame True {
              n244 = stacked-sequence {
                tunnel: w723 -> [w729 w751]
                tunnel: w722 -> [w728 _]
                tunnel: w721 -> [w727 w750]
                tunnel: w720 -> [w726 w749]
                tunnel: w719 -> [w725 _]
                tunnel: w718 -> [w724 w752]
                frame #0 {
                  n245 = while {
                    tunnel: w729 -> [w741]
                    tunnel: w728 -> [w740]
                    tunnel: w727 -> [w739]
                    tunnel: w726 -> [w738]
                    tunnel: w725 -> [w735]
                    tunnel: w724 -> [w731]
                    i -> [w742]
                    stop <- w737 stop-if-true
                    n246 = Add(x=1, y=w742) -> (x+y=w734:i32)
                    n247 = Subtract(x=w735, y=w734) -> (x-y=→"Pos X INV":dbl)
                    n248 = Divide(x=w738, y=w741) -> (x/y=w747:dbl)
                    n249 = To Double Precision Float(number=w738) -> (double precision float=w745:dbl)
                    n250 = To Double Precision Float(number=w747) -> (double precision float=w744:dbl)
                    n251 = Bundle(w745, w744) -> (w746:cluster{dbl, dbl})  [unwired: 1 out]
                    n252 = call <vilib>:"Sawtooth Waveform.vi"("sampling info"=w746, "phase"=w739, "amplitude"=w740, "frequency"=w741) -> ("signal out"=w733:waveform(dbl))  [unwired: 3 in, 4 out]
                    n253 = Multiply(x=w731, y=w733) -> (x*y=w732:waveform(dbl))
                    n254 = Equal?(x=w734, y=w735) -> (x = y?=w737:bool)
                    n255 = Subtract(x=w732, y=w740) -> (x-y=w730:waveform(dbl))
                    n256 = call "go to  Inv X"("data"=w730) -> ()  [unwired: 5 in, 14 out]
                  }
                }
                frame #1 {
                  w748 = 0
                  n257 = Divide(x=w749, y=w751) -> (x/y=w759:dbl)
                  n258 = To Double Precision Float(number=w749) -> (double precision float=w757:dbl)
                  n259 = To Double Precision Float(number=w759) -> (double precision float=w756:dbl)
                  n260 = Bundle(w757, w756) -> (w758:cluster{dbl, dbl})  [unwired: 1 out]
                  n261 = call <vilib>:"Sawtooth Waveform.vi"("sampling info"=w758, "phase"=w750, "amplitude"=w748, "frequency"=w751) -> ("signal out"=w755:waveform(dbl))  [unwired: 3 in, 4 out]
                  n262 = Multiply(x=w752, y=w755) -> (x*y=w754:waveform(dbl))
                  n263 = Subtract(x=w754, y=w748) -> (x-y=w753:waveform(dbl))
                  n264 = call "go to  Inv X2"("data"=w753) -> ()  [unwired: 5 in, 14 out]
                }
              }
            }
          }
        }
        frame #1 {
          n265 = case shown="True" w762 {
            tunnel: [w769 0] -> w760
            tunnel: w761 -> [w769 _]
            frame False {
            }
            frame True {
            }
          }
          n266 = Not Equal?(x=w760, y=w761) -> (x != y?=w768:bool)
          n267 = case shown="False" w768 {
            tunnel: w767 -> [_ w776]
            tunnel: w766 -> [_ w775]
            tunnel: w765 -> [_ w774]
            tunnel: w764 -> [_ w773]
            tunnel: w761 -> [_ w772]
            tunnel: w763 -> [_ w771]
            frame False {
            }
            frame True {
              n268 = while {
                tunnel: w776 -> [w788]
                tunnel: w775 -> [w787]
                tunnel: w774 -> [w786]
                tunnel: w773 -> [w785]
                tunnel: w772 -> [w779]
                tunnel: w771 -> [w781]
                i -> [w789]
                stop <- w784 stop-if-true
                n269 = Add(x=1, y=w789) -> (x+y=w778:i32)
                n270 = Subtract(x=w779, y=w778) -> (x-y=→"pos Y INV":dbl)
                n271 = Divide(x=w785, y=w788) -> (x/y=w794:dbl)
                n272 = To Double Precision Float(number=w785) -> (double precision float=w792:dbl)
                n273 = To Double Precision Float(number=w794) -> (double precision float=w791:dbl)
                n274 = Bundle(w792, w791) -> (w793:cluster{dbl, dbl})  [unwired: 1 out]
                n275 = call <vilib>:"Sawtooth Waveform.vi"("sampling info"=w793, "phase"=w786, "amplitude"=w787, "frequency"=w788) -> ("signal out"=w782:waveform(dbl))  [unwired: 3 in, 4 out]
                n276 = Multiply(x=w781, y=w782) -> (x*y=w783:waveform(dbl))
                n277 = Equal?(x=w778, y=w779) -> (x = y?=w784:bool)
                n278 = Add(x=w783, y=w787) -> (x+y=w777:waveform(dbl))
                n279 = call "Go to inv Y"("data"=w777) -> ()  [unwired: 5 in, 14 out]
              }
            }
          }
        }
        frame #2 {
          n280 = case shown="False" w795 {
            tunnel: [w804 0] -> w797
            tunnel: w796 -> [w804 _]
            frame False {
            }
            frame True {
            }
          }
          n281 = Not Equal?(x=w797, y=w796) -> (x != y?=w803:bool)
          n282 = case shown="True" w803 {
            tunnel: w802 -> [_ w811]
            tunnel: w801 -> [_ w810]
            tunnel: w800 -> [_ w809]
            tunnel: w799 -> [_ w808]
            tunnel: w796 -> [_ w807]
            tunnel: w798 -> [_ w806]
            frame False {
            }
            frame True {
              n283 = while {
                tunnel: w811 -> [w823]
                tunnel: w810 -> [w822]
                tunnel: w809 -> [w821]
                tunnel: w808 -> [w820]
                tunnel: w807 -> [w813]
                tunnel: w806 -> [w814]
                i -> [w824]
                stop <- w819 stop-if-true
                n284 = Add(x=1, y=w824) -> (x+y=w817:i32)
                n285 = Divide(x=w820, y=w823) -> (x/y=w829:dbl)
                n286 = To Double Precision Float(number=w820) -> (double precision float=w827:dbl)
                n287 = Subtract(x=w813, y=w817) -> (x-y=→"Pos Z inv":dbl)
                n288 = To Double Precision Float(number=w829) -> (double precision float=w826:dbl)
                n289 = Bundle(w827, w826) -> (w828:cluster{dbl, dbl})  [unwired: 1 out]
                n290 = call <vilib>:"Sawtooth Waveform.vi"("sampling info"=w828, "phase"=w821, "amplitude"=w822, "frequency"=w823) -> ("signal out"=w816:waveform(dbl))  [unwired: 3 in, 4 out]
                n291 = Multiply(x=w814, y=w816) -> (x*y=w815:waveform(dbl))
                n292 = Equal?(x=w817, y=w813) -> (x = y?=w819:bool)
                n293 = Subtract(x=w815, y=w822) -> (x-y=w812:waveform(dbl))
                n294 = call "Go to INV Z"("data"=w812) -> ()  [unwired: 4 in, 15 out]
              }
            }
          }
        }
      }
    }
  }
  "?" <- "Forward"
  "?" <- "Forward"
